vi "setScriptEventList.vi"(8 "error in (no error)":errorcluster, 10 "TScriptEventList":refnum<class "ScriptEventList.lvclass">, 11 "DataPointScript.lvclass in":refnum<class "DataPointScript.lvclass">) -> (0 "error out":errorcluster, 3 "DataPointScript.lvclass out":refnum<class "DataPointScript.lvclass">)   [LabVIEW 2011, in "Tools.lvlib" / "Scripting.lvlib" / "DataPointScript.lvclass"]
uses:
  DataPointScript.lvclass
  ScriptingEvent/ScriptEventList/ScriptEventList.lvclass
  DataPointScript.lvclass/DataPointScript.ctl
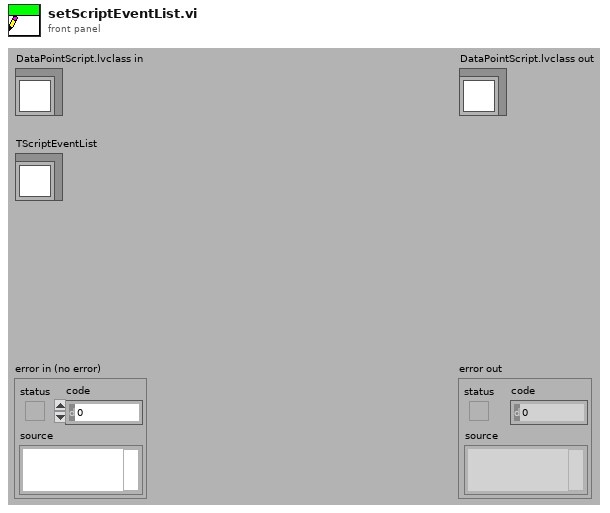
[diagram p1: front panel]
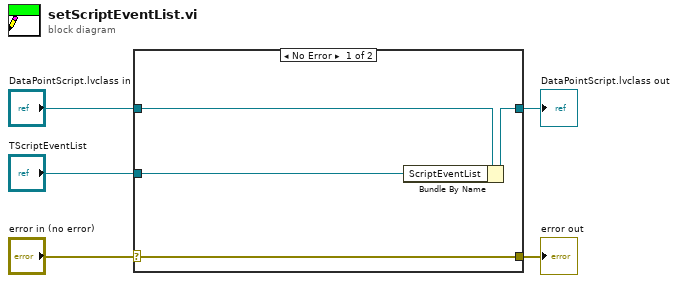
[diagram p0: block diagram]
diagram:
  n1 = case shown="No Error" "error in (no error)" {
    selector: "error in (no error)" -> [w9 w10]
    tunnel: [w9 w10] -> w4
    tunnel: [w7 w11] -> w2
    tunnel: "DataPointScript.lvclass in" -> [w8 w11]
    tunnel: "TScriptEventList" -> [w6 _]
    frame No Error {
      n2 = Bundle By Name(cluster=w8, "ScriptEventList"=w6) -> (w7:refnum<class "DataPointScript.lvclass">)
    }
    frame Error {
    }
  }
  "error out" <- w4
  "DataPointScript.lvclass out" <- w2
